vi "GetUpdatePanel.vi"(1 "Tab Control":T1(ring)) -> (0 "Numeric":u32)   [LabVIEW 2009]
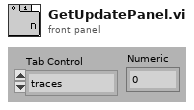
[diagram p1: front panel]
types:
  T1 = enum32{"traces", "coincidence settings", "liftetime settings", "autcorrelation", "F2-Bursts"}
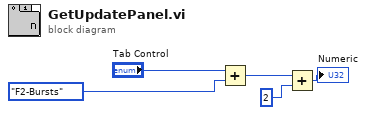
[diagram p0: block diagram]
diagram:
  n1 = Add(x="Tab Control", y=T1."F2-Bursts") -> (x+y=w4:u32)
  n2 = Add(x=w4, y=u32 2) -> (x+y=→"Numeric":u32)
